vi "BinarizationRegistration.vi"(8 "error in":errorcluster, 11 "Image cluster in":T2) -> (0 "error out":errorcluster, 1 "quality":dbl, 2 "x translation":i32, 3 "Image cluster out":T2)   [LabVIEW 2012]
uses:
  <vilib>/vision/Image Controls.llb/IMAQ Image.ctl
  <vilib>/vision/NI_Vision_Development_Module.lvlib
panel:
  out "aligned false color":T1(plugin-control)
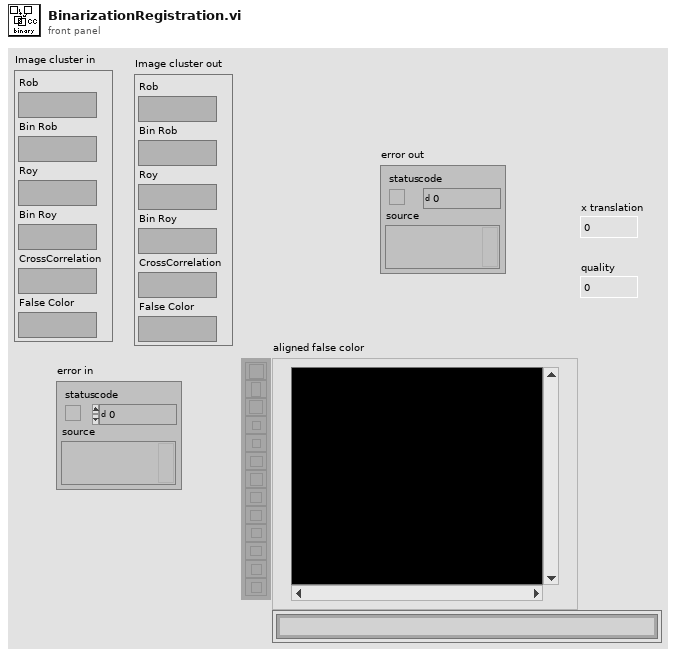
[diagram p1: front panel]
types:
  T1 = typedef "IMAQ Image.ctl" = refnum<image>
  T2 = cluster{"Rob":T1, "Bin Rob":T1, "Roy":T1, "Bin Roy":T1, "CrossCorrelation":T1, "False Color":T1}
  T3 = cluster{"Lower value":sgl, "Upper value":sgl, "Replace Value":sgl, "Keep/Replace Value (Replace)":bool}[]
  T4 = cluster{"Lower value":sgl, "Upper value":sgl, "Replace Value":sgl, "Keep/Replace Value (Replace)":bool}
  T5 = cluster{"Mean Value":sgl, "Standard Variation":sgl, "Minimal Value":sgl, "Maximal Value":sgl, "Area (calibrated)":sgl, "Area (pixels)":u32, "%":sgl, "Calibration Valid":bool}
  T6 = cluster{"Area":dbl, "Number of Holes":dbl, "Bounding Rect":cluster{"Left":dbl, "Top":dbl, "Right":dbl, "Bottom":dbl}, "Center of Mass":cluster{"X":dbl, "Y":dbl}, "Orientation":dbl, "Dimensions":cluster{"Width":dbl, "Height":dbl}}[]
  T7 = cluster{"Area":dbl, "Number of Holes":dbl, "Bounding Rect":cluster{"Left":dbl, "Top":dbl, "Right":dbl, "Bottom":dbl}, "Center of Mass":cluster{"X":dbl, "Y":dbl}, "Orientation":dbl, "Dimensions":cluster{"Width":dbl, "Height":dbl}}
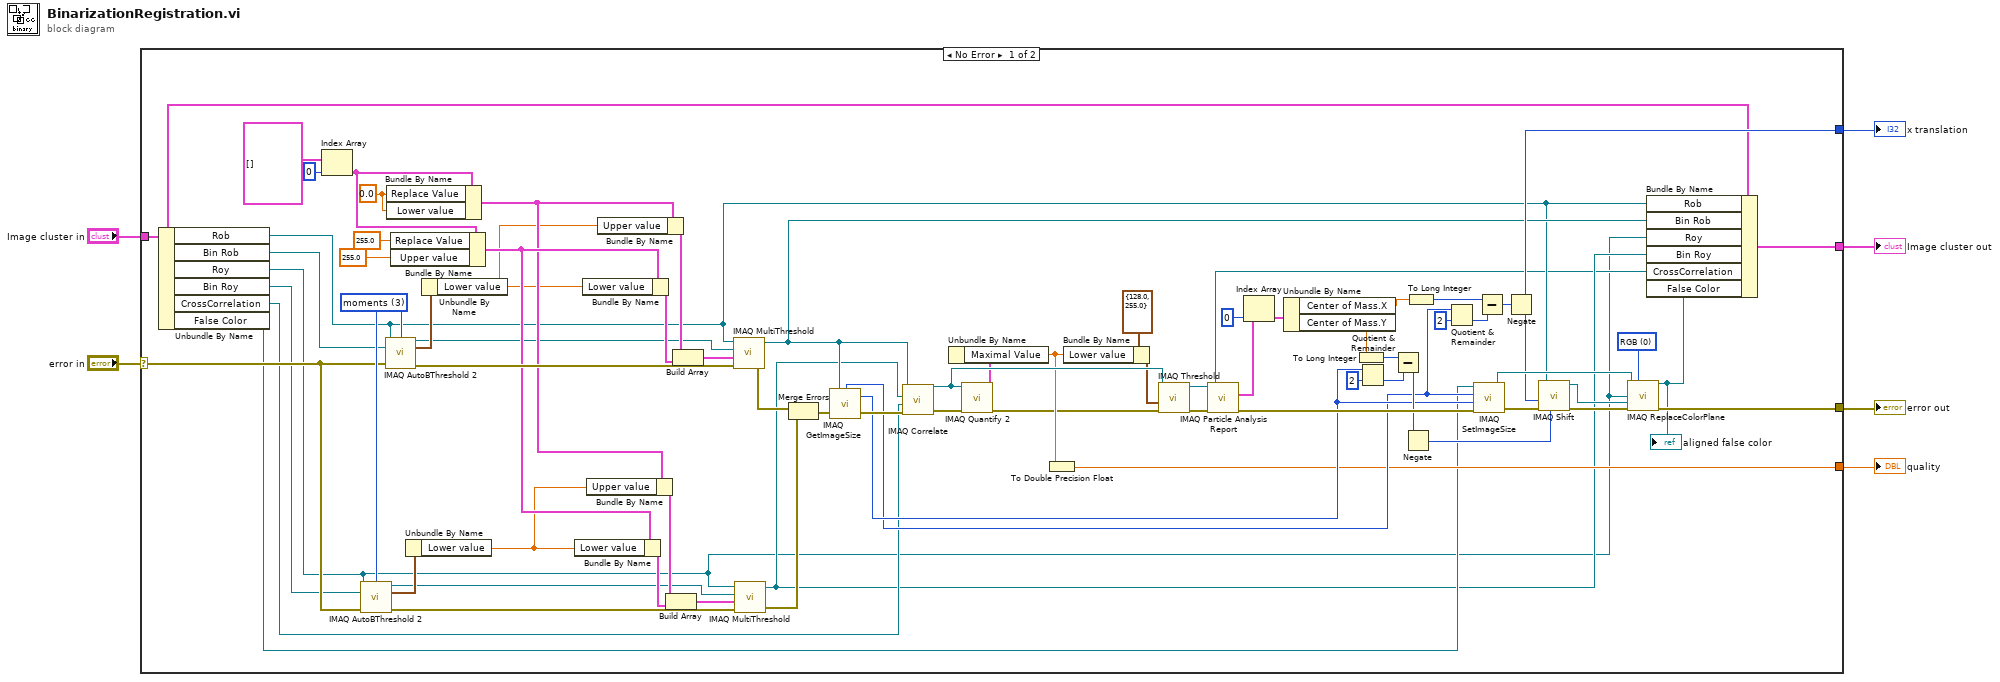
[diagram p0: block diagram]
diagram:
  n1 = case shown="No Error" "error in" {
    selector: "error in" -> [w19 w82]
    tunnel: [w51 _] -> w6
    tunnel: [w34 _] -> w5
    tunnel: [w20 w82] -> w4
    tunnel: "Image cluster in" -> [w14 w81]
    tunnel: [w7 w81] -> w1
    frame No Error {
      w61 = u16 0 items=["RGB", "HSL", "HSV", "HSI"] ("Color Mode")
      w42 = 3 items=["clustering", "entropy", "metric", "moments", "inter-class variance"] ("Method (clustering)")
      w74 = sgl 0.0 ("Replace Value")
      n2 = Unbundle By Name(w14) -> ("Rob"=w12:T1, "Bin Rob"=w18:T1, "Roy"=w8:T1, "Bin Roy"=w17:T1, "CrossCorrelation"=w16:T1, "False Color"=w15:T1)
      n3 = Index Array(array=T3 [] ("Threshold Data"), index=0) -> (element=w75:T4)
      n4 = call "IMAQ AutoBThreshold 2"("Image Src"=w8, "Method (clustering)"=w42, "Image Dst"=w17, "error in (no error)"=w19) -> ("Image Dst Out"=w53:T1, "Threshold Range Out"=w67:cluster{"Lower value":sgl, "Upper value":sgl}, "error out"=w69:errorcluster)  [unwired: 9 in]
      n5 = call "IMAQ AutoBThreshold 2"("Image Src"=w12, "Method (clustering)"=w42, "Image Dst"=w18, "error in (no error)"=w19) -> ("Image Dst Out"=w52:T1, "Threshold Range Out"=w78:cluster{"Lower value":sgl, "Upper value":sgl}, "error out"=w77:errorcluster)  [unwired: 9 in]
      n6 = Bundle By Name(cluster=w75, "Replace Value"=w74, "Lower value"=w74) -> (w65:T4)
      n7 = Bundle By Name(cluster=w75, "Replace Value"=sgl 255.0, "Upper value"=sgl 255.0) -> (w66:T4)
      n8 = Unbundle By Name(w67) -> ("Lower value"=w36:sgl)
      n9 = Unbundle By Name(w78) -> ("Lower value"=w35:sgl)
      n10 = Bundle By Name(cluster=w66, "Lower value"=w36) -> (w63:T4)
      n11 = Bundle By Name(cluster=w66, "Lower value"=w35) -> (w71:T4)
      n12 = Bundle By Name(cluster=w65, "Upper value"=w36) -> (w64:T4)
      n13 = Bundle By Name(cluster=w65, "Upper value"=w35) -> (w72:T4)
      n14 = Build Array(w64, w63) -> (w68:T3)
      n15 = Build Array(w72, w71) -> (w70:T3)
      n16 = call "IMAQ MultiThreshold"("error in (no error)"=w77, "Threshold Data"=w70, "Image Dst"=w52, "Image Src"=w12) -> ("error out"=w40:errorcluster, "Image Dst Out"=w13:T1)  [unwired: 1 in]
      n17 = call "IMAQ MultiThreshold"("error in (no error)"=w69, "Threshold Data"=w68, "Image Dst"=w53, "Image Src"=w8) -> ("error out"=w41:errorcluster, "Image Dst Out"=w11:T1)  [unwired: 1 in]
      n18 = Merge Errors(w40, w41) -> (w21:errorcluster)
      n19 = call "IMAQ GetImageSize"("Image"=w13, "error in (no error)"=w21) -> ("Y Resolution"=w38:i32, "X Resolution"=w37:i32, "error out"=w39:errorcluster)  [unwired: 2 in]
      n20 = call "IMAQ Correlate"("Image Src"=w13, "Image Template"=w11, "Image Dst"=w16, "error in (no error)"=w39) -> ("Image Dst Out"=w54:T1, "error out"=w58:errorcluster)  [unwired: 3 in]
      n21 = call "IMAQ Quantify 2"("error in (no error)"=w58, "Image"=w54) -> ("error out"=w31:errorcluster, "Global Report"=w32:T5)  [unwired: 7 in, 1 out]
      n22 = Unbundle By Name(w32) -> ("Maximal Value"=w33:sgl)
      n23 = To Double Precision Float(number=w33) -> (double precision float=w34:dbl)
      n24 = Bundle By Name(cluster=cluster{"Lower value":sgl, "Upper value":sgl} {"Lower value"=128.0, "Upper value"=255.0} ("Range"), "Lower value"=w33) -> (w29:cluster{"Lower value":sgl, "Upper value":sgl})
      n25 = call "IMAQ Threshold"("error in (no error)"=w31, "Range"=w29, "Image Src"=w54) -> ("error out"=w27:errorcluster, "Image Dst Out"=w28:T1)  [unwired: 7 in]
      n26 = call "IMAQ Particle Analysis Report"("error in (no error)"=w27, "Image"=w28) -> ("error out"=w57:errorcluster, "Particle Reports (Pixels)"=w22:T6, "Image Out (duplicate)"=w10:T1)  [unwired: 4 in, 3 out]
      n27 = Index Array(array=w22, index=0) -> (element=w25:T7)
      n28 = Unbundle By Name(w25) -> ("Center of Mass.X"=w24:dbl, "Center of Mass.Y"=w23:dbl)
      n29 = To Long Integer(number=w23) -> (32bit integer=w56:i32)
      n30 = Quotient & Remainder(x=w38, y=2) -> (floor(x/y)=w46:i32)  [unwired: 1 out]
      n31 = Subtract(x=w56, y=w46) -> (x-y=w47:i32)
      n32 = Negate(x=w47) -> (-x=w50:i32)
      n33 = To Long Integer(number=w24) -> (32bit integer=w48:i32)
      n34 = Quotient & Remainder(x=w37, y=2) -> (floor(x/y)=w43:i32)  [unwired: 1 out]
      n35 = call "IMAQ SetImageSize"("error in (no error)"=w57, "Y Resolution"=w38, "X Resolution"=w37, "Image"=w15) -> ("error out"=w59:errorcluster, "Image Out"=w60:T1)  [unwired: 1 in]
      n36 = Subtract(x=w48, y=w43) -> (x-y=w49:i32)
      n37 = Negate(x=w49) -> (-x=w51:i32)
      n38 = call "IMAQ Shift"("YOffset"=w50, "error in (no error)"=w59, "XOffset"=w51, "Image Src"=w12) -> ("error out"=w62:errorcluster, "Image Dst Out"=w55:T1)  [unwired: 6 in]
      n39 = call "IMAQ ReplaceColorPlane"("Image Src"=w60, "Color Mode"=w61, "Red or Hue Plane"=w8, "Green or Sat Plane"=w55, "error in (no error)"=w62) -> ("Image Dst Out"=w9:T1, "error out"=w20:errorcluster)  [unwired: 9 in]
      "aligned false color" <- w9
      n40 = Bundle By Name(cluster=w14, "Rob"=w12, "Bin Rob"=w13, "Roy"=w8, "Bin Roy"=w11, "CrossCorrelation"=w10, "False Color"=w9) -> (w7:T2)
    }
    frame Error {
    }
  }
  "error out" <- w4
  "x translation" <- w6
  "quality" <- w5
  "Image cluster out" <- w1
